vi "read station ps rem sense config.vi"(8 "error in":errorcluster, 10 "station":string, 11 "configuration file path in":path) -> (0 "error out":errorcluster, 2 "enable remote sense":bool, 3 "configuration file path out":path)   [LabVIEW 2018]
uses:
  05.UserVI's/file io/ini/type defs/ini file actions.ctl
  05.UserVI's/file io/ini/type defs/ini entry value.ctl
  05.UserVI's/file io/ini/type defs/ini entry types.ctl
  05.UserVI's/file io/ini/type defs/ini entry.ctl
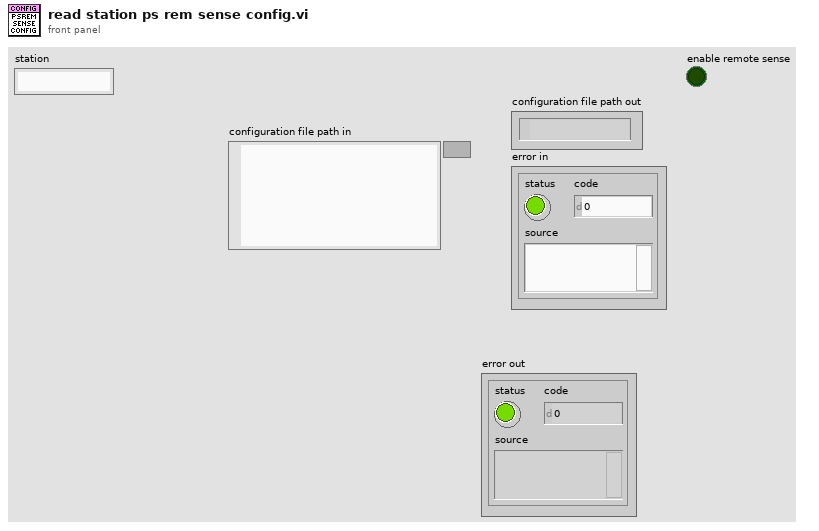
[diagram p1: front panel]
types:
  T1 = typedef "ini entry value.ctl" = cluster{"Boolean":bool, "Dbl":dbl, "I32":i32, "Path":path, "String":string, "U32":u32}
  T2 = typedef "ini file actions.ctl" = enum16{"read ini", "write ini"}
  T3 = typedef "ini entry.ctl" = cluster{"section":string, "key":string, "type":T4, "default value":T1}
  T4 = typedef "ini entry types.ctl" = enum16{"Boolean", "Double", "I32", "Path", "String", "U32"}
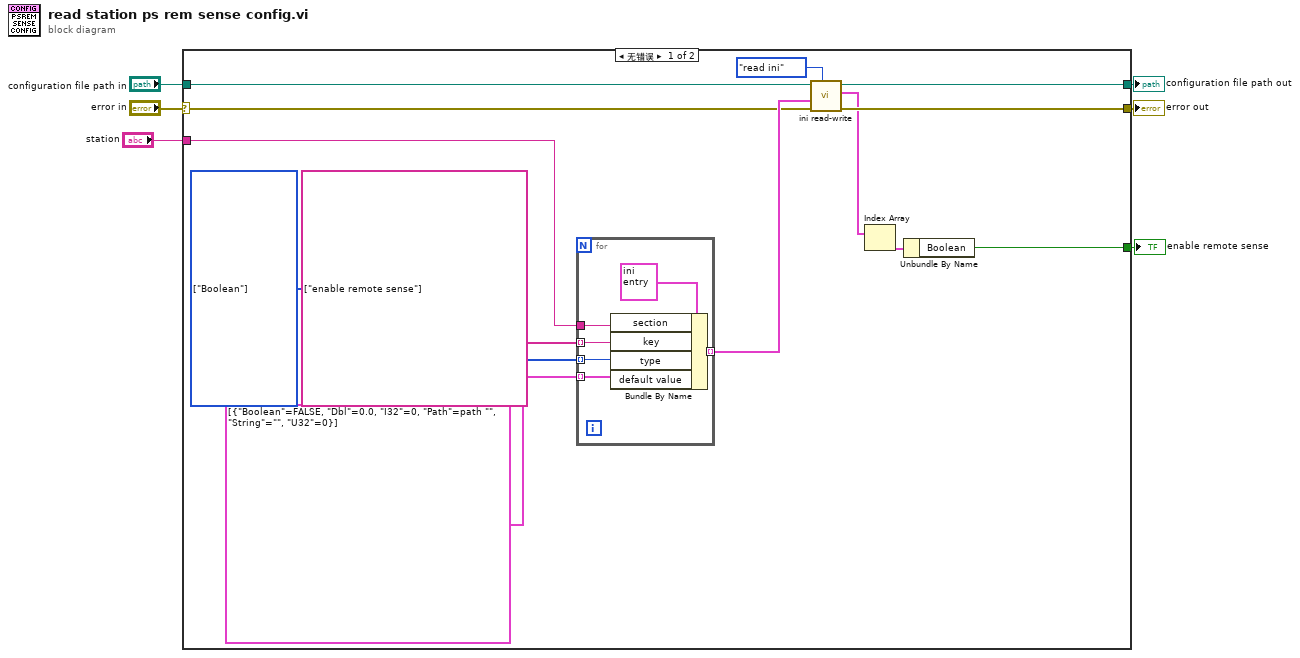
[diagram p0: block diagram]
diagram:
  n1 = case shown="无错误" "error in" {
    selector: "error in" -> [w12 w27]
    tunnel: "configuration file path in" -> [w19 w26]
    tunnel: [w17 w26] -> w5
    tunnel: [w11 w27] -> w4
    tunnel: "station" -> [w10 _]
    tunnel: [w7 _] -> w1
    frame No Error {
      w15 = T4[] [enum."Boolean"] items=["Boolean", "Double", "I32", "Path", "String", "U32"]
      n2 = for {
        tunnel: w10 -> [w24]
        tunnel: string[] ["enable remote sense"] -> [w23] mode=indexing
        tunnel: w15 -> [w22] mode=indexing
        tunnel: T1[] [{"Boolean"=FALSE, "Dbl"=0.0, "I32"=0, "Path"=path "", "String"="", "U32"=0}] -> [w21] mode=indexing
        tunnel: [w20] -> w13 mode=indexing
        n3 = Bundle By Name(cluster=T3 {"section"="", "key"="", "type"=enum."Boolean", "default value"={"Boolean"=FALSE, "Dbl"=0.0, "I32"=0, "Path"=path "", "String"="", "U32"=0}}, "section"=w24, "key"=w23, "type"=w22, "default value"=w21) -> (w20:T3)
      }
      n4 = call "ini read-write.vi"("action"=ini_file_actions."read ini", "error in (no error)"=w12, "ini entry descriptors"=w13, "configuration file path"=w19) -> ("error out"=w11:errorcluster, "values out"=w9:T1[], "configuration file path out"=w17:path)  [unwired: 5 in]
      n5 = Index Array(array=w9) -> (element=w8:T1)  [unwired: 1 in]
      n6 = Unbundle By Name(w8) -> ("Boolean"=w7:bool)
    }
    frame Error {
    }
  }
  "configuration file path out" <- w5
  "error out" <- w4
  "enable remote sense" <- w1
